vi "Actor Core.vi"(8 "error in":errorcluster, 11 "Nested in":refnum<class "BD_CAFÉ_MXN_ENG.lvclass">) -> (0 "error out":errorcluster, 3 "Actor out":refnum<class "Actor.lvclass">)   [LabVIEW 2019, in "BD_CAFÉ_MXN_ENG.lvlib" / "BD_CAFÉ_MXN_ENG.lvclass"]
doc: "(<B>Filename</B>: Actor Framework.lvlib:Actor.lvclass:Actor Core.vi)\n\nReceives messages to the actor, reacts to them, and initiates any error handling that may shut the actor down.\n\nDescendant classes may override this VI to append parallel tasks for the actor to complete while it handles messages. Overrides use the Call Parent Method node."
uses:
  <vilib>/ActorFramework/Actor/Actor.lvclass
  <vilib>/ActorFramework/Stop Msg/Stop Msg.lvclass
  C:/Program Files (x86)/National Instruments/LabVIEW 2019/vi.lib/ActorFramework/Actor/Actor.lvclass
panel:
  in  "COMPRAR MERCANCÍA":bool
  in  "10 PESOS MEXICANOS":bool
  in  "5 PESOS MEXICANOS":bool
  in  "2 PESOS MEXICANOS":bool
  in  "1 PESO MEXICANO":bool
  in  "SOLICITAR MERCANCIA":bool
  out "PRECIO":dbl
  out "CANTIDAD":dbl
  out "PRODUCTO":string
  out "MONEDA":string
  in  "MERCANCÍA":i32(listbox)
  out "CRÉDITO":dbl
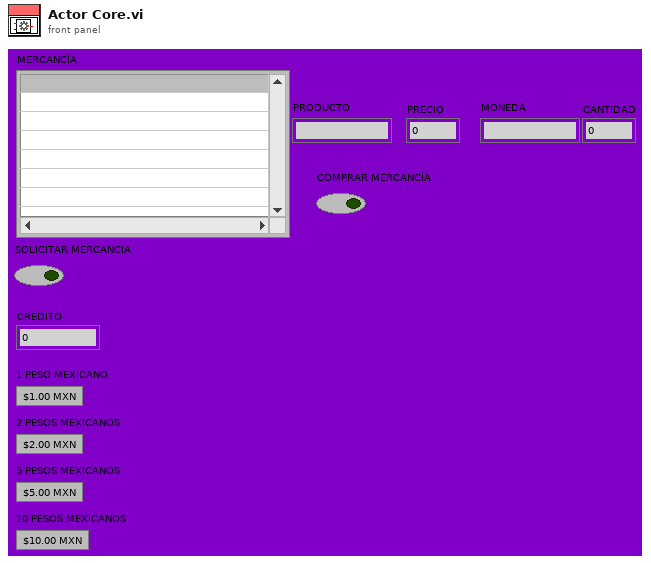
[diagram p1: front panel]
types:
  T1 = cluster{"CANTIDAD":dbl, "MONEDA":string, "PRECIO ":dbl, "PRODUCTO":string}
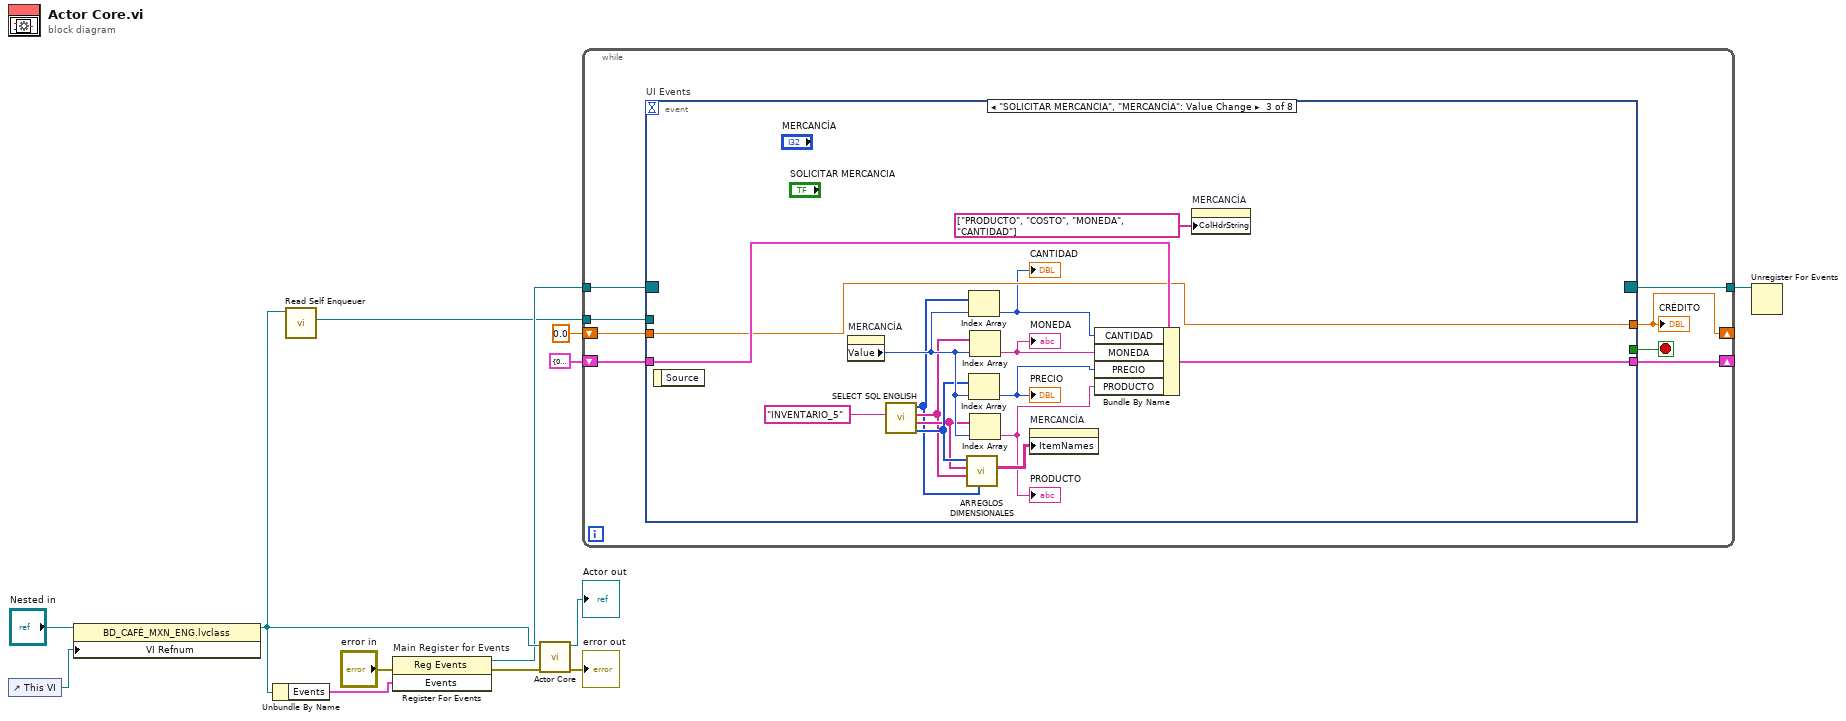
[diagram p0: block diagram]
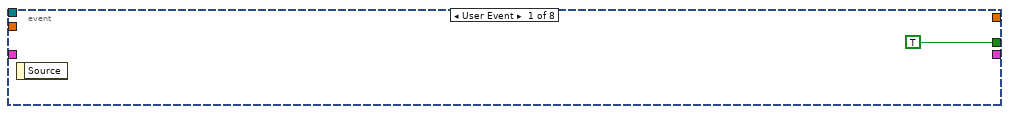
[diagram p2: hidden frame]
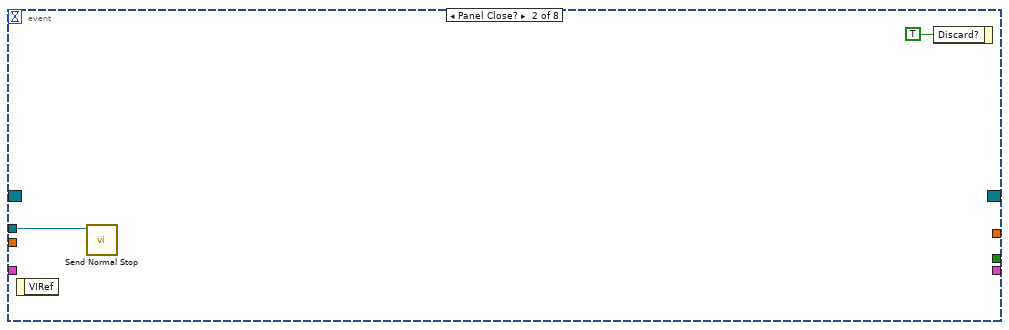
[diagram p3: hidden frame]
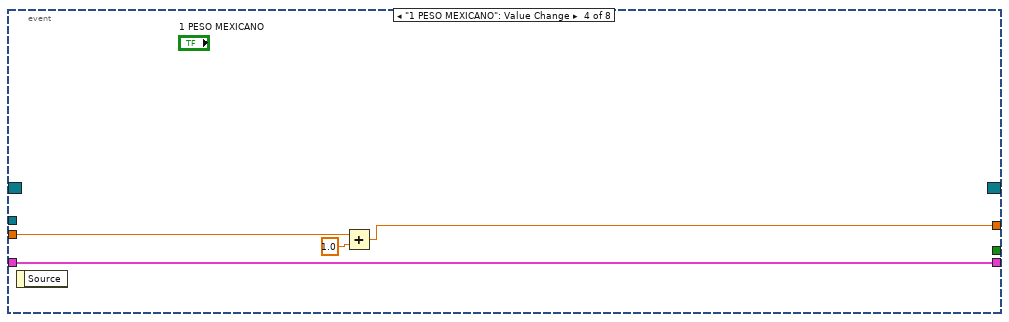
[diagram p4: hidden frame]
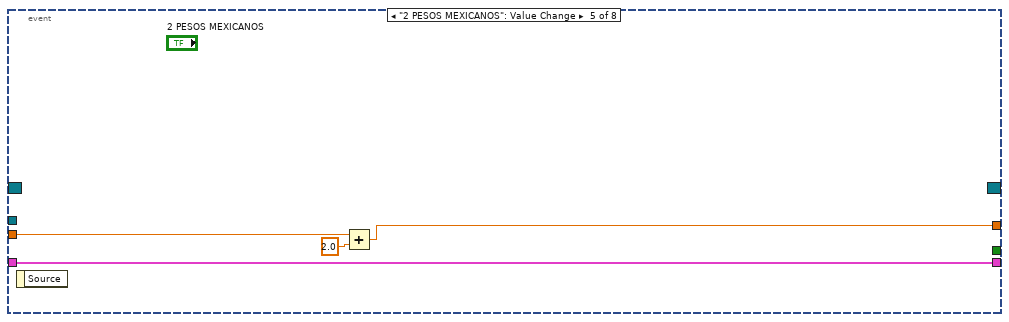
[diagram p5: hidden frame]
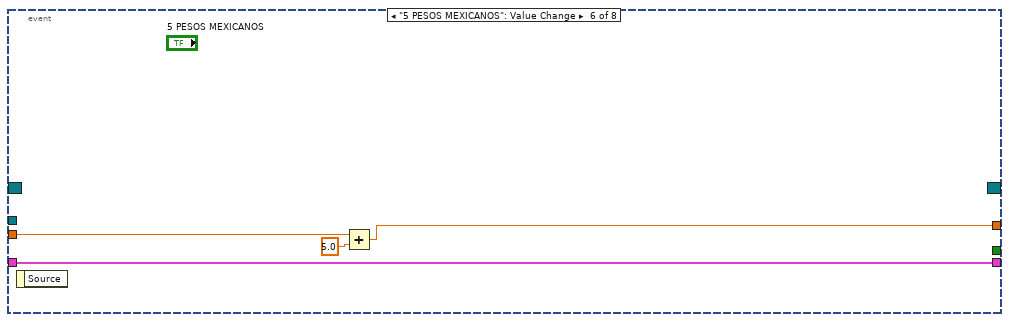
[diagram p6: hidden frame]
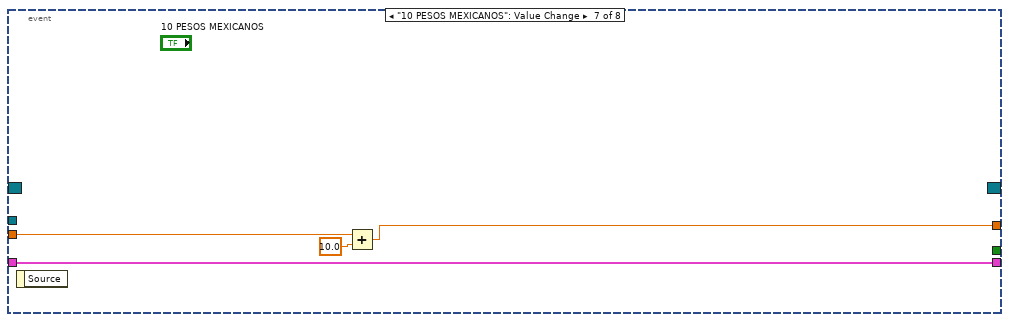
[diagram p7: hidden frame]
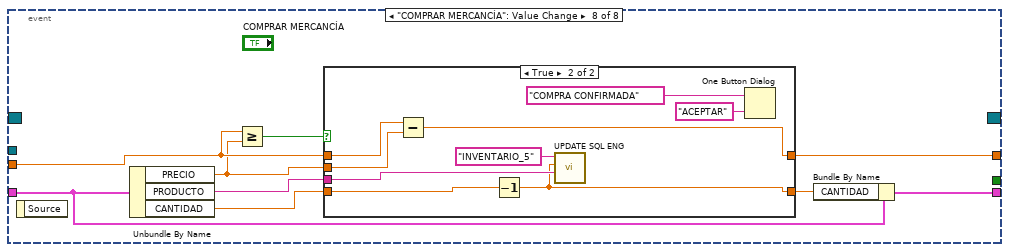
[diagram p8: hidden frame]
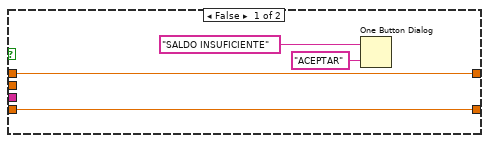
[diagram p9: hidden frame]
diagram:
  n1 = control-ref of="This VI"() -> (w6:refnum<vi>)
  n2 = property class="BD_CAFÉ_MXN_ENG.lvclass"(reference="Nested in", "VI Refnum"=w6) -> (reference out=w7:refnum<class "BD_CAFÉ_MXN_ENG.lvclass">)  [unwired: 1 in, 1 out]
  n3 = Unbundle By Name(w7) -> ("Events"=w11:cluster{"Stop":refnum<user-event>})
  n4 = call <vilib>:"Read Self Enqueuer.vi"("Actor"=w7) -> ("Self Enqueuer"=w2:refnum<class "Message Enqueuer.lvclass">)  [unwired: 10 in]
  n5 = register-events "Main Register for Events"(error in="error in", w11) -> (reference out=w3:refnum<event-registration>, error out=w8:errorcluster)  [unwired: 1 in]
  n6 = call-parent "Actor Core.vi"("error in"=w8, "Actor in"=w7) -> ("error out"=→"error out":errorcluster, "Actor out"=→"Actor out":refnum<class "Actor.lvclass">)  [unwired: 8 in]
  n7 = while {
    tunnel: w3 -> [w21]
    tunnel: [w19] -> w1
    tunnel: w2 -> [w18]
    shift-right: [w16] -> _
    shift-left: T1 {"CANTIDAD"=0.0, "MONEDA"="", "PRECIO "=0.0, "PRODUCTO"=""} -> [w17]
    shift-right: [w14] -> _
    shift-left: 0.0 -> [w15]
    stop <- w20 stop-if-true
    n8 = event "UI Events" shown="[2] \"SOLICITAR MERCANCIA\", \"MERCANCÍA\": Value Change" {
      selector: w21 -> [_ _ _ _ _ _ _ _]
      dyn-events: [_ _ _ _ _ _ _ _] -> w19
      timeout: _ -> [_ _ _ _ _ _ _ _]
      tunnel: [TRUE _ _ _ _ _ _ _] -> w20
      tunnel: w18 -> [_ w23 _ _ _ _ _ _]
      tunnel: w17 -> [_ _ w37 w43 w47 w51 w55 w64]
      tunnel: [_ _ w36 w43 w47 w51 w55 w60] -> w16
      tunnel: [_ _ w34 w40 w44 w48 w52 w56] -> w14
      tunnel: w15 -> [_ _ w34 w42 w46 w50 w54 w58]
      event User Event {
        n9 = event-data() -> ()  [unwired: 1 in, 1 out]
      }
      event Panel Close? {
        n10 = event-data() -> ()  [unwired: 1 in, 1 out]
        n11 = call <vilib>:"Send Normal Stop.vi"("Message Enqueuer"=w23) -> ()  [unwired: 10 in, 1 out]
        n12 = event-data("Discard?"=TRUE) -> ()  [unwired: 1 in, 1 out]
      }
      event "SOLICITAR MERCANCIA", "MERCANCÍA": Value Change {
        n13 = event-data() -> ()  [unwired: 1 in, 1 out]
        n14 = property on="MERCANCÍA" class="MCListbox (strict)"() -> ("Value"=w35:i32)  [unwired: 2 in, 2 out]
        n15 = call "SELECT SQL ENGLISH.vi"("INVENTARIO"="INVENTARIO_5") -> ("COSTO"=w32:i64[], "PRODUCTO"=w31:string[], "MONEDA"=w30:string[], "CANTIDAD"=w29:i64[])  [unwired: 7 in]
        n16 = call "ARREGLOS DIMENSIONALES.vi"("CANTIDAD"=w29, "MONEDA"=w30, "PRODUCTO"=w31, "COSTO"=w32) -> ("Array"=w38:string[][])  [unwired: 7 in]
        n17 = Index Array(array=w29, index=w35) -> (element=w28:i64)
        "CANTIDAD" <- w28
        n18 = Index Array(array=w32, index=w35) -> (element=w26:i64)
        "PRECIO" <- w26
        n19 = Index Array(array=w30, index=w35) -> (element=w27:string)
        "MONEDA" <- w27
        n20 = Index Array(array=w31, index=w35) -> (element=w25:string)
        "PRODUCTO" <- w25
        n21 = property on="MERCANCÍA" class="MCListbox (strict)"("ItemNames"=w38) -> ()  [unwired: 2 in, 2 out]
        n22 = Bundle By Name(cluster=w37, "CANTIDAD"=w28, "MONEDA"=w27, "PRECIO"=w26, "PRODUCTO"=w25) -> (w36:T1)
        n23 = property on="MERCANCÍA" class="MCListbox (strict)"("ColHdrString"=string[] ["PRODUCTO", "COSTO", "MONEDA", "CANTIDAD"] ("Column Header Strings[]")) -> ()  [unwired: 2 in, 2 out]
      }
      event "1 PESO MEXICANO": Value Change {
        n24 = event-data() -> ()  [unwired: 1 in, 1 out]
        n25 = Add(x=w42, y=1.0) -> (x+y=w40:dbl)
      }
      event "2 PESOS MEXICANOS": Value Change {
        n26 = event-data() -> ()  [unwired: 1 in, 1 out]
        n27 = Add(x=w46, y=2.0) -> (x+y=w44:dbl)
      }
      event "5 PESOS MEXICANOS": Value Change {
        n28 = event-data() -> ()  [unwired: 1 in, 1 out]
        n29 = Add(x=w50, y=5.0) -> (x+y=w48:dbl)
      }
      event "10 PESOS MEXICANOS": Value Change {
        n30 = event-data() -> ()  [unwired: 1 in, 1 out]
        n31 = Add(x=w54, y=10.0) -> (x+y=w52:dbl)
      }
      event "COMPRAR MERCANCÍA": Value Change {
        n32 = event-data() -> ()  [unwired: 1 in, 1 out]
        n33 = Unbundle By Name(w64) -> ("PRECIO"=w57:dbl, "PRODUCTO"=w61:string, "CANTIDAD"=w62:dbl)
        n34 = Greater Or Equal?(x=w58, y=w57) -> (x >= y?=w63:bool)
        n35 = case shown="True" w63 {
          tunnel: w62 -> [w67 w75]
          tunnel: w61 -> [_ w70]
          tunnel: [w67 w69] -> w59
          tunnel: w58 -> [w68 w74]
          tunnel: w57 -> [_ w73]
          tunnel: [w68 w72] -> w56
          frame False {
            n36 = One Button Dialog(message="SALDO INSUFICIENTE", button name ("OK")="ACEPTAR") -> ()  [unwired: 1 out]
          }
          frame True {
            n37 = Subtract(x=w74, y=w73) -> (x-y=w72:dbl)
            n38 = Decrement(x=w75) -> (x-1=w69:dbl)
            n39 = call "UPDATE SQL ENG.vi"("PRODUCTO"=w70, "number"=w69, "TABLA"="INVENTARIO_5") -> ()  [unwired: 9 in]
            n40 = One Button Dialog(message="COMPRA CONFIRMADA", button name ("OK")="ACEPTAR") -> ()  [unwired: 1 out]
          }
        }
        n41 = Bundle By Name(cluster=w64, "CANTIDAD"=w59) -> (w60:T1)
      }
    }
    "CRÉDITO" <- w14
  }
  n42 = Unregister For Events(event registration refnum=w1) -> ()  [unwired: 1 in, 1 out]
